vi "QMH Template.vi"() -> ()   [LabVIEW 2013, in "AMC.lvlib"]
uses:
  AMC.lvlib
panel:
  out "Status":string
  in  "Process":bool
  in  "Exit":bool
  in  "State Variables":cluster{"CurrentFile":path}
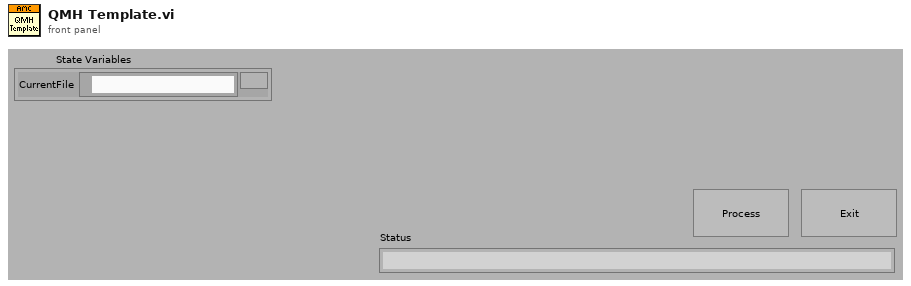
[diagram p1: front panel]
types:
  T1 = typedef "AMC.lvlib/Message Queue.ctl" = refnum<queue>
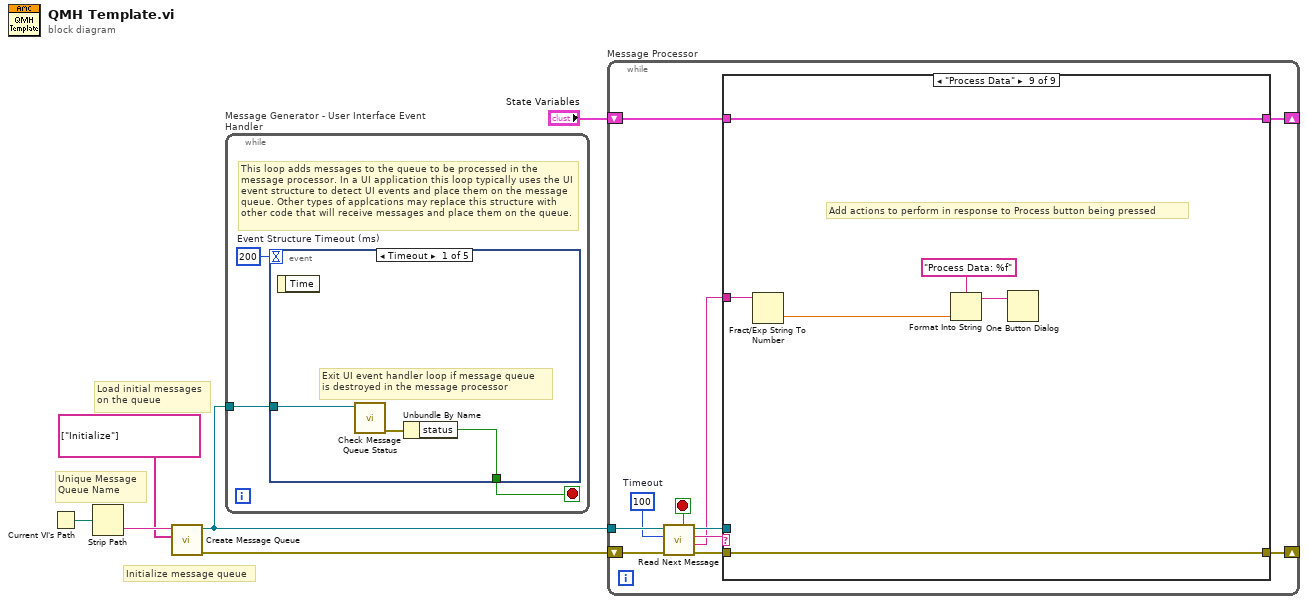
[diagram p0: block diagram]
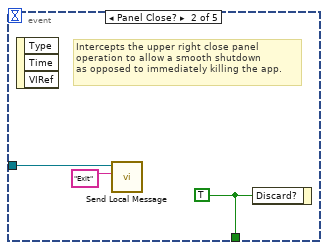
[diagram p2: hidden frame]
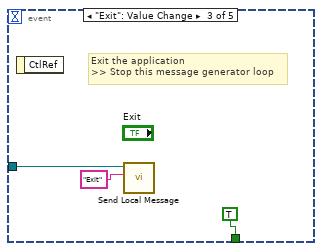
[diagram p3: hidden frame]
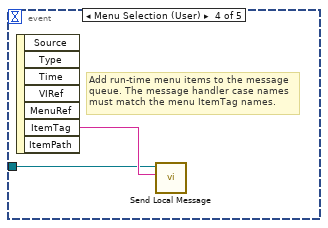
[diagram p4: hidden frame]
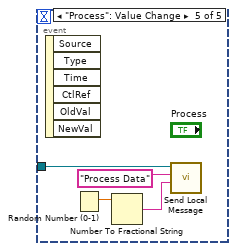
[diagram p5: hidden frame]
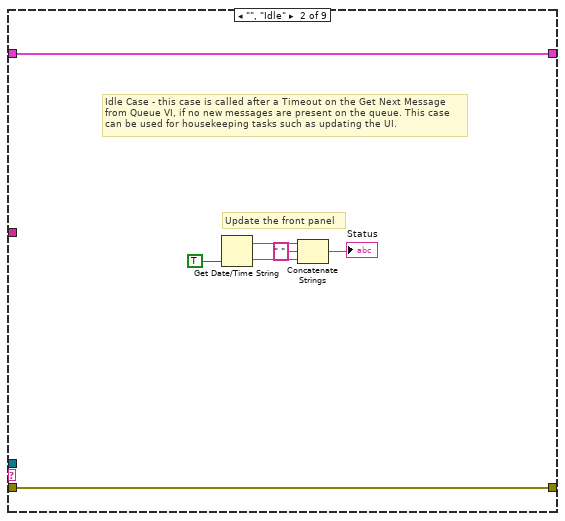
[diagram p7: hidden frame]
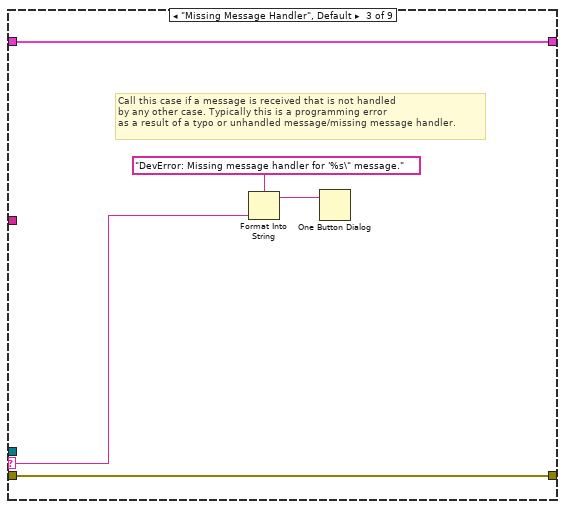
[diagram p8: hidden frame]
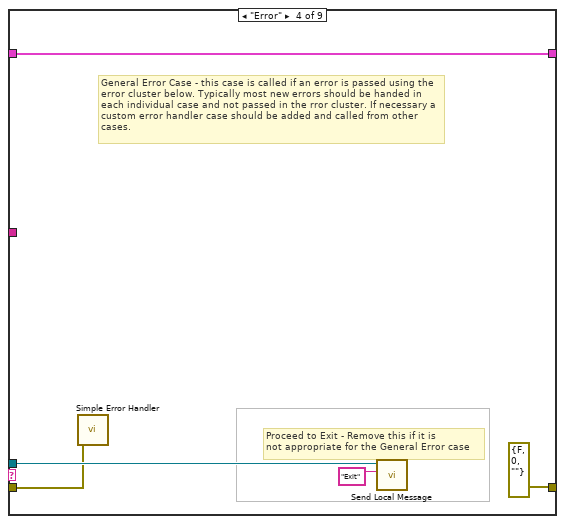
[diagram p9: hidden frame]
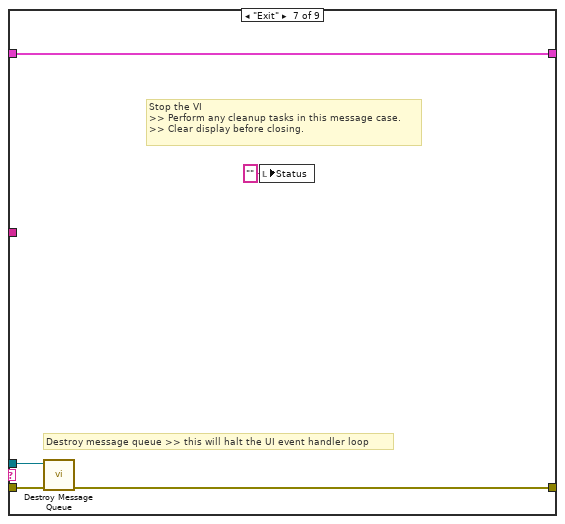
[diagram p12: hidden frame]
diagram:
  # "Initialize message queue"
  # "Unique Message\nQueue Name"
  # "Load initial messages\non the queue"
  n1 = Current VI's Path() -> (path=w6:path)
  n2 = Strip Path(path=w6) -> (name=w2:string)  [unwired: 1 out]
  n3 = call "Create Message Queue.vi"("Initial Message Names"=string[] ["Initialize"], "Message Queue Name"=w2) -> ("error out"=w4:errorcluster, "Message Queue out"=w3:T1)  [unwired: 2 in, 6 out]
  n4 = while "Message Generator - User Interface Event Handler" {
    tunnel: w3 -> [w7]
    stop <- w8 stop-if-true
    w9 = 200  # Event Structure Timeout (ms)
    # "This loop adds messages to the queue to be processed in the message processor. In a UI application this loop typically uses the UI event structure to detect UI events and place them on the message queue. Other types of applcations may replace this structure with other code that will receive messages and place them on the queue."
    n5 = event shown="[0] Timeout" {
      selector: _ -> [_ _ _ _ _]
      dyn-events: _ -> [_ _ _ _ _]
      timeout: w9 -> [_ _ _ _ _]
      tunnel: [w10 w15 TRUE ("Discard?") _ _] -> w8
      tunnel: w7 -> [w11 w13 w16 w19 w24]
      event Timeout {
        # "Exit UI event handler loop if message queue\nis destroyed in the message processor"
        n6 = event-data() -> ()  [unwired: 2 out]
        n7 = call "Check Message Queue Status.vi"("Message queue in"=w11) -> ("error out"=w12:errorcluster)  [unwired: 7 in, 2 out]
        n8 = Unbundle By Name(w12) -> ("status"=w10:bool)
      }
      event Panel Close? {
        w15 = TRUE ("Discard?")
        # "Intercepts the upper right close panel\noperation to allow a smooth shutdown\nas opposed to immediately killing the app."
        n9 = event-data() -> ()  [unwired: 4 out]
        n10 = call "Send Local Message.vi"("Message Name"="Exit", "Message Queue in"=w13) -> ()  [unwired: 4 in, 6 out]
        n11 = event-data("Discard?"=w15) -> ()  [unwired: 1 in, 1 out]
      }
      event "Exit": Value Change {
        # "Exit the application\n>> Stop this message generator loop"
        n12 = event-data() -> ()  [unwired: 2 out]
        n13 = call "Send Local Message.vi"("Message Name"="Exit", "Message Queue in"=w16) -> ()  [unwired: 4 in, 6 out]
      }
      event Menu Selection (User) {
        # "Add run-time menu items to the message\nqueue. The message handler case names must match the menu ItemTag names."
        n14 = event-data() -> ("ItemTag"=w20:string)  [unwired: 7 out]
        n15 = call "Send Local Message.vi"("Message Name"=w20, "Message Queue in"=w19) -> ()  [unwired: 4 in, 6 out]
      }
      event "Process": Value Change {
        n16 = event-data() -> ()  [unwired: 7 out]
        n17 = Random Number (0-1)() -> (number: 0 to 1=w21:dbl)
        n18 = Number To Fractional String(number=w21) -> (F-format string=w22:string)  [unwired: 3 out]
        n19 = call "Send Local Message.vi"("Message Value"=w22, "Message Name"="Process Data", "Message Queue in"=w24) -> ()  [unwired: 3 in, 6 out]
      }
    }
  }
  n20 = while "Message Processor" {
    shift-left: w4 -> [w29]
    shift-right: [w33] -> _
    tunnel: w3 -> [w30]
    shift-left: "State Variables" -> [w35]
    shift-right: [w34] -> _
    stop <- w32 stop-if-true
    w27 = 100  # Timeout
    n21 = call "Read Next Message.vi"("error in (no error)"=w29, "timeout (1ms)"=w27, "Message Queue in"=w30) -> ("error out"=w28:errorcluster, "Message Value"=w25:string, "Message Name"=w26:string, "Message Queue out"=w31:T1, "Exit Process"=w32:bool)  [unwired: 2 in, 2 out]
    n22 = case shown="\"Process Data\"" w26 {
      selector: w26 -> [_ _ w47 _ _ _ _ _ _]
      tunnel: [w37 w44 w49 w54 w56 w58 w63 w65 w70] -> w34
      tunnel: w35 -> [w37 w44 w49 w54 w56 w58 w63 w65 w70]
      tunnel: w31 -> [_ _ _ w52 _ _ w60 _ _]
      tunnel: w28 -> [w36 w43 w48 w50 w55 w57 w61 w64 w71]
      tunnel: [w36 w43 w48 errorcluster {"status"=FALSE, "code"=0, "source"=""} ("error out") w55 w57 w59 w64 w71] -> w33
      tunnel: w25 -> [_ _ _ _ _ _ _ _ w69]
      frame "---------- Framework Operations ----------" {
        # "Dummy case to add a seperator in the Case Structure menu"
      }
      frame "", "Idle" {
        # "Update the front panel"
        # "Idle Case - this case is called after a Timeout on the Get Next Message from Queue VI, if no new messages are present on the queue. This case can be used for housekeeping tasks such as updating the UI."
        n23 = Get Date/Time String(want seconds? (F)=TRUE) -> (date string=w42:string, time string=w41:string)  [unwired: 2 out]
        n24 = Concatenate Strings(w42, " " ("string"), w41) -> (→"Status":string)
      }
      frame "Missing Message Handler", Default {
        # "Call this case if a message is received that is not handled \nby any other case. Typically this is a programming error\nas a result of a typo or unhandled message/missing message handler."
        n25 = Format Into String(format string="DevError: Missing message handler for '%s\" message." ("message"), w47) -> (resulting string=w45:string)  [unwired: 2 in, 1 out]
        n26 = One Button Dialog(message=w45) -> ()  [unwired: 2 out]
      }
      frame "Error" {
        # "Proceed to Exit - Remove this if it is\nnot appropriate for the General Error case"
        # "General Error Case - this case is called if an error is passed using the error cluster below. Typically most new errors should be handed in each individual case and not passed in the rror cluster. If necessary a custom error handler case should be added and called from other cases."
        n27 = call <vilib>:"Simple Error Handler.vi"("error in (no error)"=w50) -> ()  [unwired: 1 in, 8 out]
        n28 = call "Send Local Message.vi"("Message Name"="Exit", "Message Queue in"=w52) -> ()  [unwired: 4 in, 6 out]
      }
      frame "---------- Generic Operations ----------" {
        # "Dummy case to add a seperator in the Case Structure menu"
      }
      frame "Initialize" {
        # "Initialize the state variables and user interface"
      }
      frame "Exit" {
        # "Destroy message queue >> this will halt the UI event handler loop"
        # "Stop the VI\n>> Perform any cleanup tasks in this message case.\n>> Clear display before closing."
        n29 = call "Destroy Message Queue.vi"("error in (no error)"=w61, "Message Queue in"=w60) -> ("error out"=w59:errorcluster)  [unwired: 9 out]
        n30 = local write "Status"("" ("Status")) -> ()
      }
      frame "---------- Application Operations ----------" {
        # "Dummy case to add a seperator in the Case Structure menu"
      }
      frame "Process Data" {
        # "Add actions to perform in response to Process button being pressed"
        n31 = Fract/Exp String To Number(string=w69) -> (number=w68:dbl)  [unwired: 4 out]
        n32 = Format Into String(format string="Process Data: %f" ("message"), w68) -> (resulting string=w66:string)  [unwired: 2 in, 1 out]
        n33 = One Button Dialog(message=w66) -> ()  [unwired: 2 out]
      }
    }
  }
